vi "MakeExternalDisplay-1.vi"(5 "[IN] WxH":cluster{"Width":i32, "Height":i32}, 6 "[IN] Resize to Img Size?":bool=TRUE, 7 "[IN] # Window":i32, 8 "error IN":errorcluster, 11 "[IN] Image":T1) -> (0 "error OUT":errorcluster)   [LabVIEW 2020]
uses:
  <vilib>/vision/Image Controls.llb/IMAQ Image.ctl
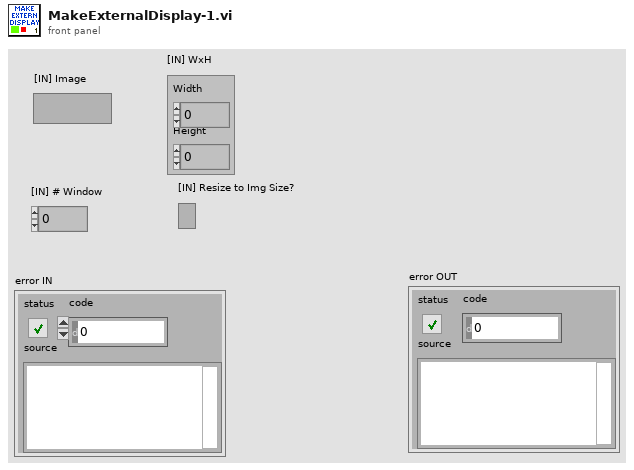
[diagram p1: front panel]
types:
  T1 = typedef "IMAQ Image.ctl" = refnum<image>
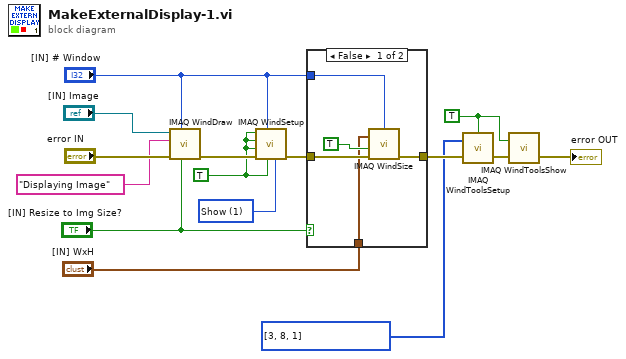
[diagram p0: block diagram]
diagram:
  w1 = 1 items=["Hide", "Show", "No change"] ("Scrollbars (No change)")
  w2 = u32[] [3, 8, 1] items=["No Selection", "Point", "Line", "Rectangle", "Oval", "Polygon", "Freehand Region", "Annulus", "Zoom", "Pan", "Broken Line", "Freehand Line", "Rotated Rectangle"] ("Tools")
  w5 = TRUE ("Show Coordinates? (T)")
  w11 = TRUE ("Window is floating? (No)")
  n1 = call "IMAQ WindDraw"("Resize to Image Size? (Y)"="[IN] Resize to Img Size?", "Window Number (0...15)"="[IN] # Window", "error in (no error)"="error IN", "Title"="Displaying Image", "Image"="[IN] Image") -> ("error out"=w12:errorcluster)  [unwired: 5 in, 1 out]
  n2 = call "IMAQ WindSetup"("Scrollbars (No change)"=w1, "Window is floating? (No)"=w11, "Window Number (0...15)"="[IN] # Window", "error in (no error)"=w12, "Window has title bar? (Yes)"=w11, "Window can close? (Yes)"=w11, "Window can grow? (Yes)"=w11) -> ("error out"=w9:errorcluster)  [unwired: 4 in]
  n3 = case shown="False" "[IN] Resize to Img Size?" {
    tunnel: w9 -> [w20 w21]
    tunnel: "[IN] # Window" -> [w18 _]
    tunnel: "[IN] WxH" -> [w17 _]
    tunnel: [w16 w21] -> w4
    frame False {
      n4 = call "IMAQ WindSize"("error in (no error)"=w20, "Scrollbars? (N)"=TRUE, "Width & Height"=w17, "Window Number"=w18) -> ("error out"=w16:errorcluster)  [unwired: 2 in, 2 out]
    }
    frame True {
    }
  }
  n5 = call "IMAQ WindToolsSetup"("Show Coordinates? (T)"=w5, "Tools"=w2, "error in (no error)"=w4) -> ("error out"=w6:errorcluster)  [unwired: 3 in]
  n6 = call "IMAQ WindToolsShow"("Hide/Show (Show)"=w5, "error in (no error)"=w6) -> ("error out"=→"error OUT":errorcluster)  [unwired: 3 in, 1 out]
